vi "Calibration.vi"(8 "Error in":errorcluster) -> (0 "Error out":errorcluster)   [LabVIEW 2022 SP3, in "Bontech Calibration.lvlib" / "Bontech Calibration.lvclass"]
uses:
  Bontech Calibration.lvclass
  TypeDef/Calibration VI States.ctl
  Bontech Calibration.lvclass/Bontech Calibration.ctl
  <vilib>/vision/Image Controls.llb/IMAQ Image.ctl
  BonTechDetector/Controls/Acquisition Modes.ctl
  BonTechDetector/Controls/Acquisition Commands.ctl
  BonTechDetector/BonTechDetector.lvlib
panel:
  in  "Calibrate":bool
  in  "Get Bright Image":bool
  in  "Get Dark Image":bool
  out "Status":string
  out "Progress":u16(slide) scale=0.0..100.0
  # "Aayvu Calibration Tool"
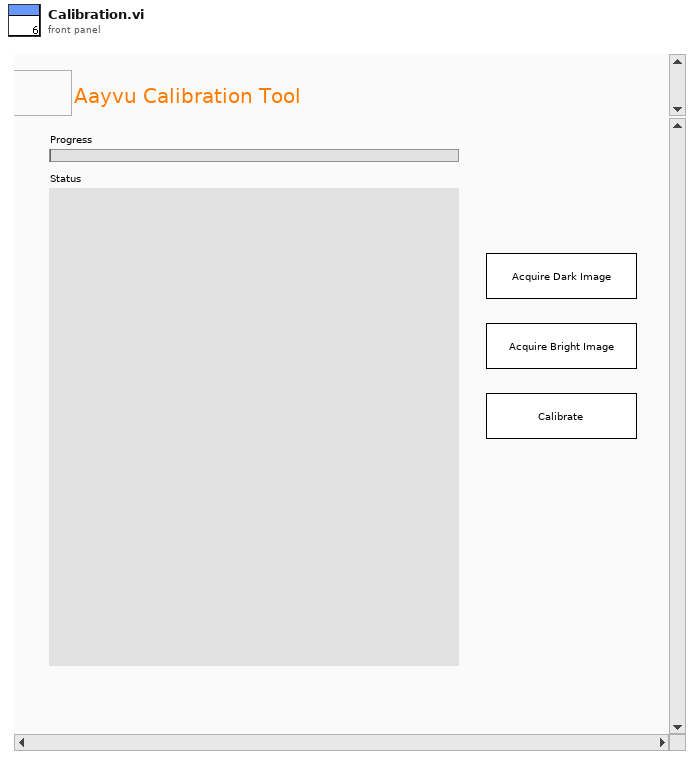
[diagram p1: front panel]
types:
  T1 = typedef "IMAQ Image.ctl" = refnum<image>
  T2 = cluster{"Status":string, "nWidth":u32, "nHeight":u32, "Save Path":string, "nSensorIP":string, "nHostIP":string, "live image":T1, "acq image":T1, "lpszSerialNum":string, "Progress":u8, "Iteration":i32, "refImg":u16[], "pImg":u16[], "Cal Dir":string, "avgBuff":dbl[], "pDarkImg":u16[], "pBrightImg":u16[]}
  T3 = cluster{"UI Ref":cluster{"Progress Ref":refnum<vi>, "Status Ref":refnum<vi>}, "Sensor Data":cluster{"nHostIP":string, "nSensorIP":string, "lpszSerialNum":string, "Cal Dir":string, "refImg":u16[], "pImg":u16[], "nHeight":u32, "nWidth":u32, "pBrightImg":u16[], "pDarkImg":u16[], "avgBuff":dbl[], "Iteration":i32, "Progress":u8, "acq image":T1, "live image":T1, "Save Path":string, "Status":string}}
  T4 = cluster{"Command":string, "Img Save Path":path, "pImg":u16[], "Iteration":i32, "Status":string}
  T5 = typedef "Calibration VI States.ctl" = enum16{"Poll", "Init", "Start Acquisition", "Acquire Dark Image", "Acquire Bright Image", "Calibrate", "Stop Acquisition", "Save Image", "Error", "Exit"}
  T6 = cluster{"nHostIP":string, "nSensorIP":string, "lpszSerialNum":string, "Cal Dir":string, "refImg":u16[], "pImg":u16[], "nHeight":u32, "nWidth":u32, "pBrightImg":u16[], "pDarkImg":u16[], "avgBuff":dbl[], "Iteration":i32, "Progress":u8, "acq image":T1, "live image":T1, "Save Path":string, "Status":string}
  T7 = typedef "BonTechDetector.lvlib/Acquisition Modes.ctl" = enum32{"IMAGECAP_TRIGGER_MODE", "IMAGECAP_AED_MODE", "IMAGECAP_SOFTTRIGGER_MODE", "IMAGECAP_AVG_COUNT_MODE", "IMAGECAP_AVG_AED_MODE", "IMAGECAP_CONTINUOUS_MODE", "IMAGECAP_VIEWER_MODE", "IMAGECAP_CONTINUOUS_BINNING_MODE"}
  T8 = typedef "Image Type" = u32
  T9 = typedef "BonTechDetector.lvlib/Acquisition Commands.ctl" = u32
  T10 = enum16{"big-endian, network order", "native, host order", "little-endian"}
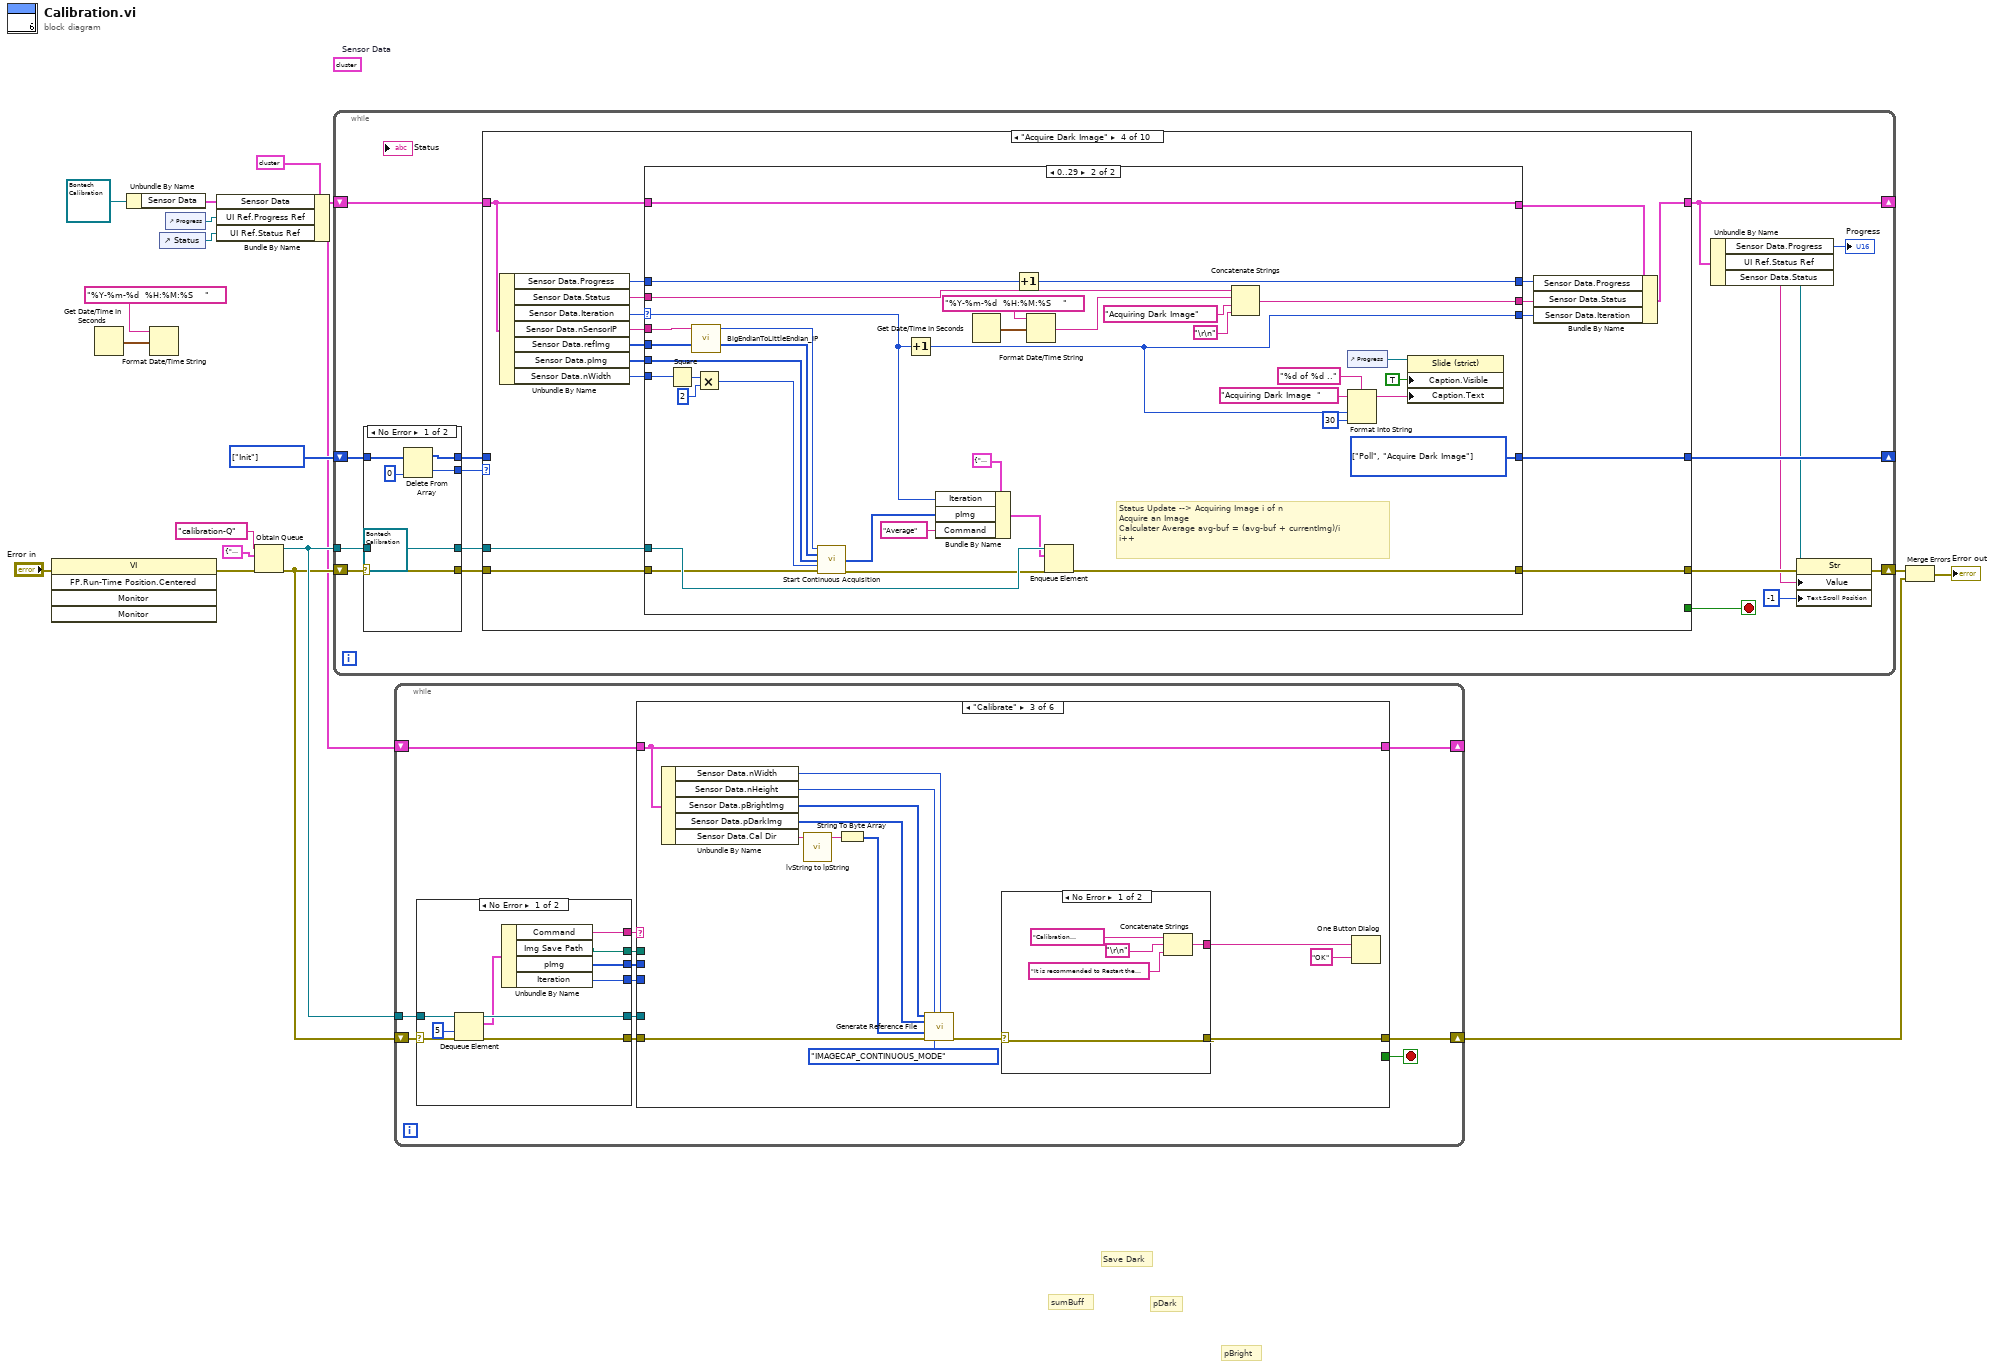
[diagram p0: block diagram]
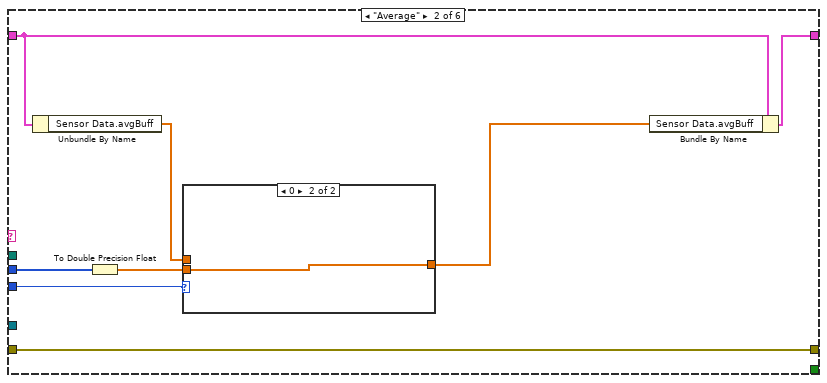
[diagram p3: hidden frame]
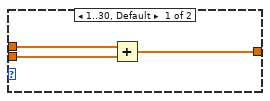
[diagram p4: hidden frame]
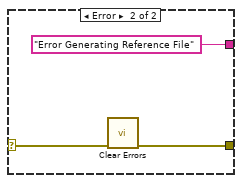
[diagram p5: hidden frame]
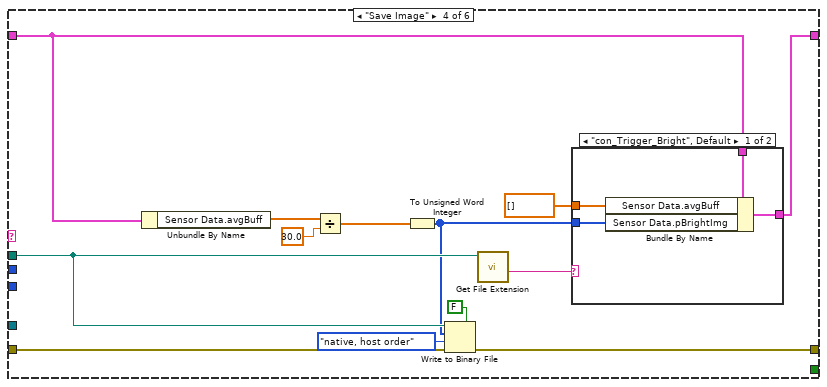
[diagram p6: hidden frame]
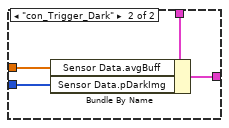
[diagram p7: hidden frame]
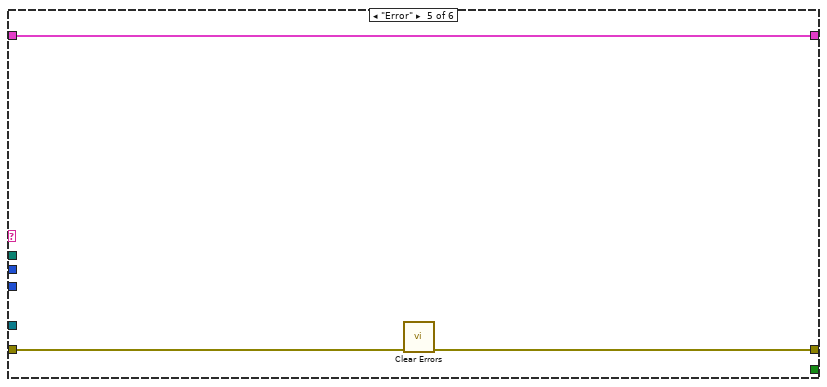
[diagram p8: hidden frame]
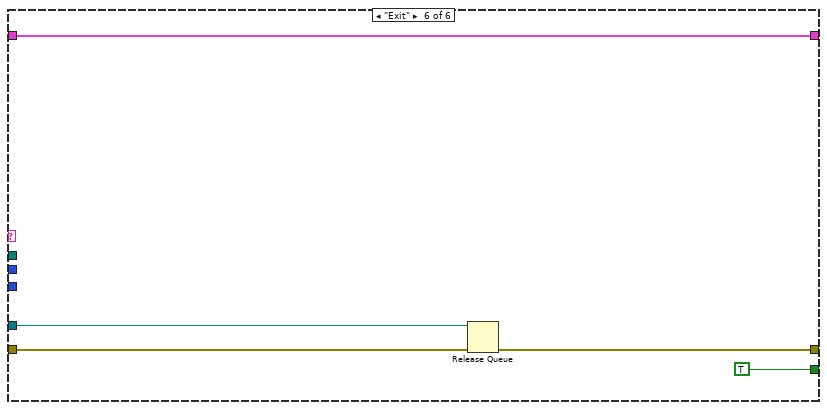
[diagram p9: hidden frame]
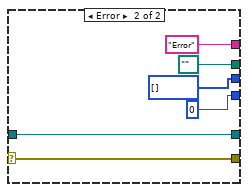
[diagram p10: hidden frame]
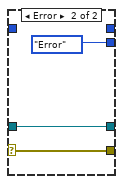
[diagram p11: hidden frame]
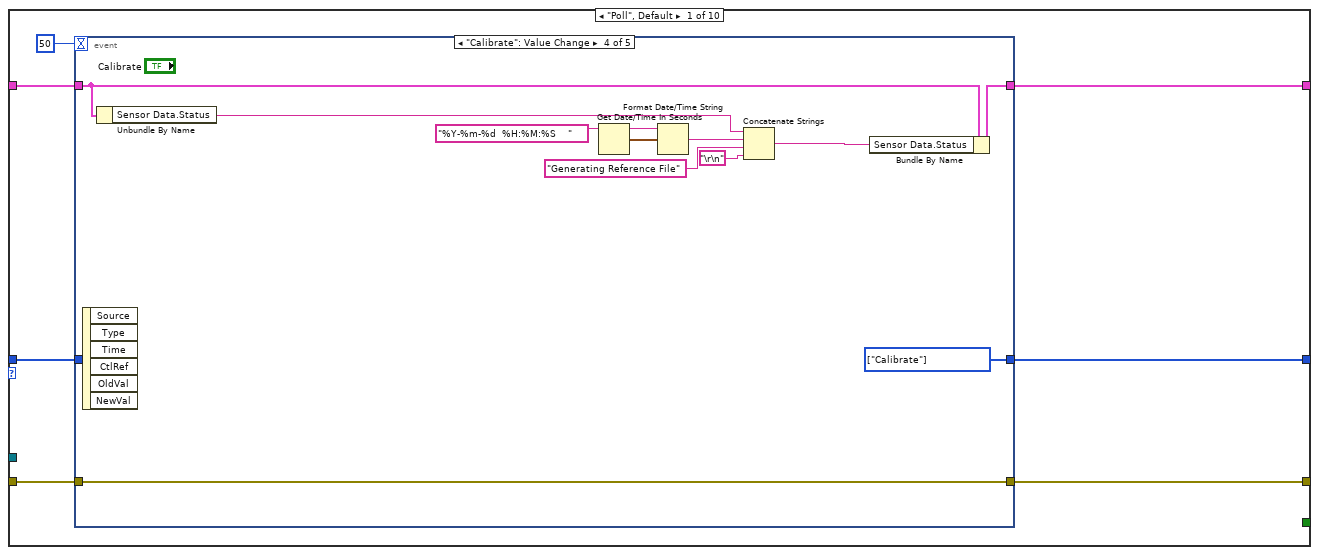
[diagram p12: hidden frame]
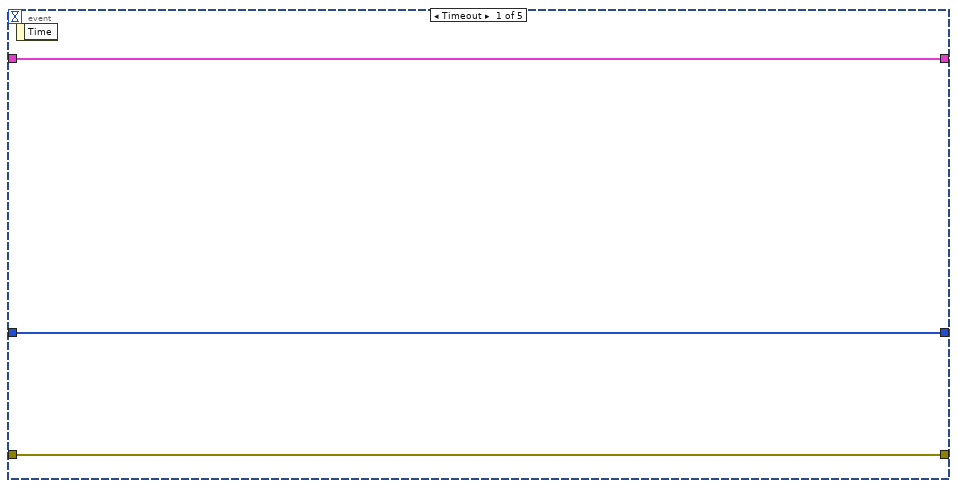
[diagram p13: hidden frame]
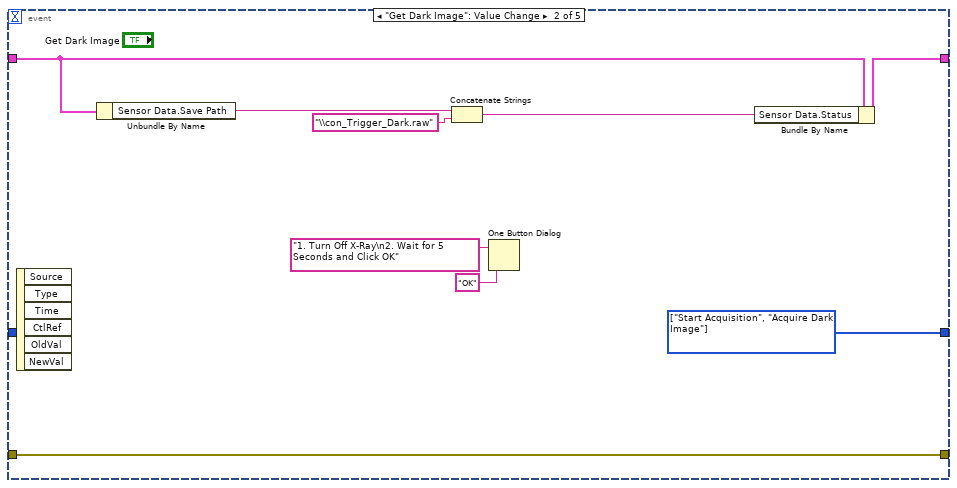
[diagram p14: hidden frame]
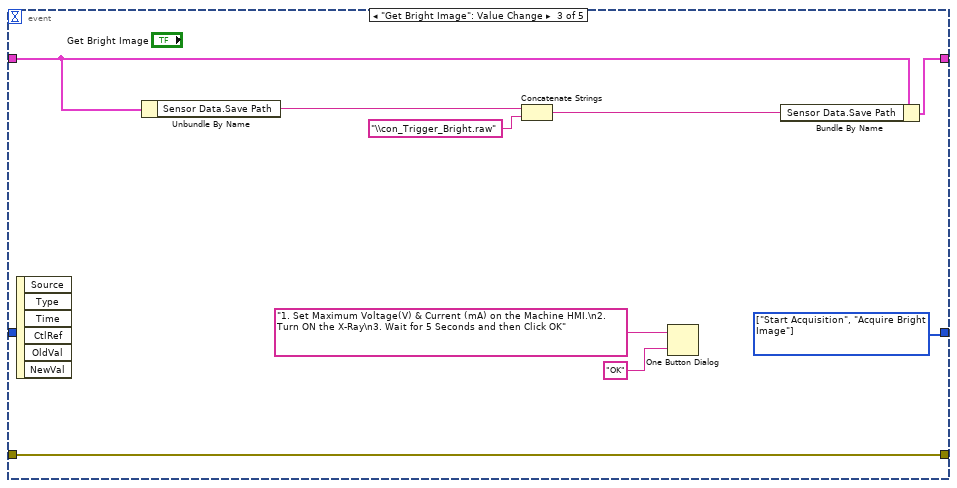
[diagram p15: hidden frame]
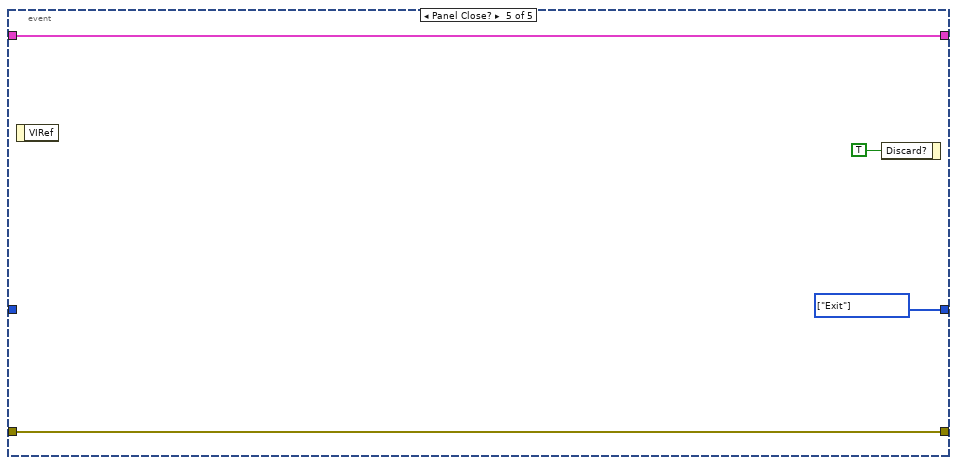
[diagram p16: hidden frame]
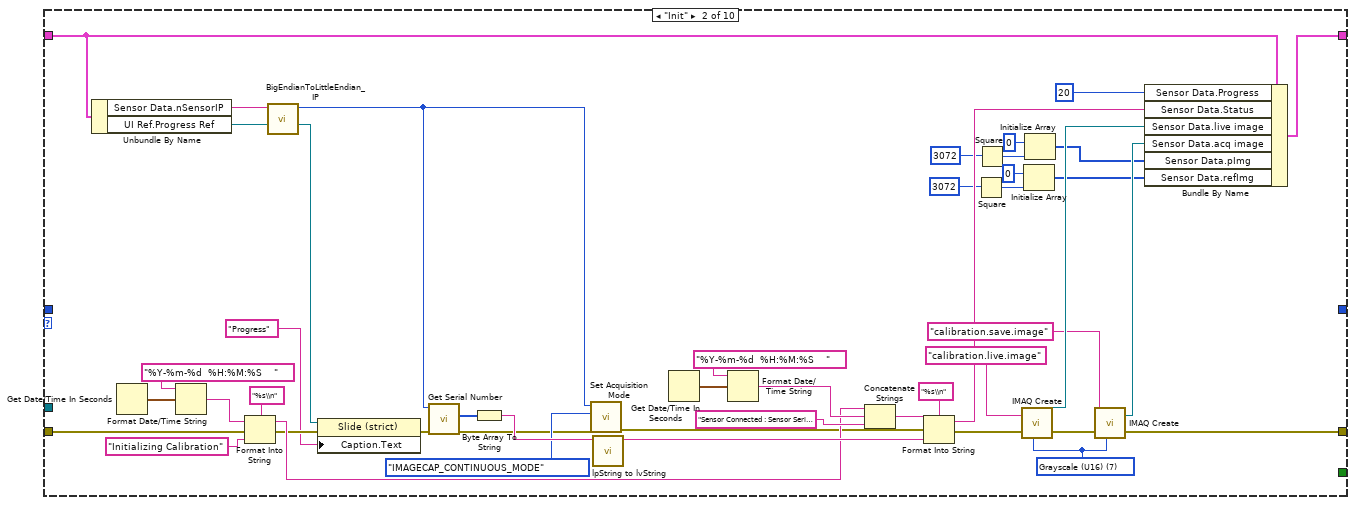
[diagram p17: hidden frame]
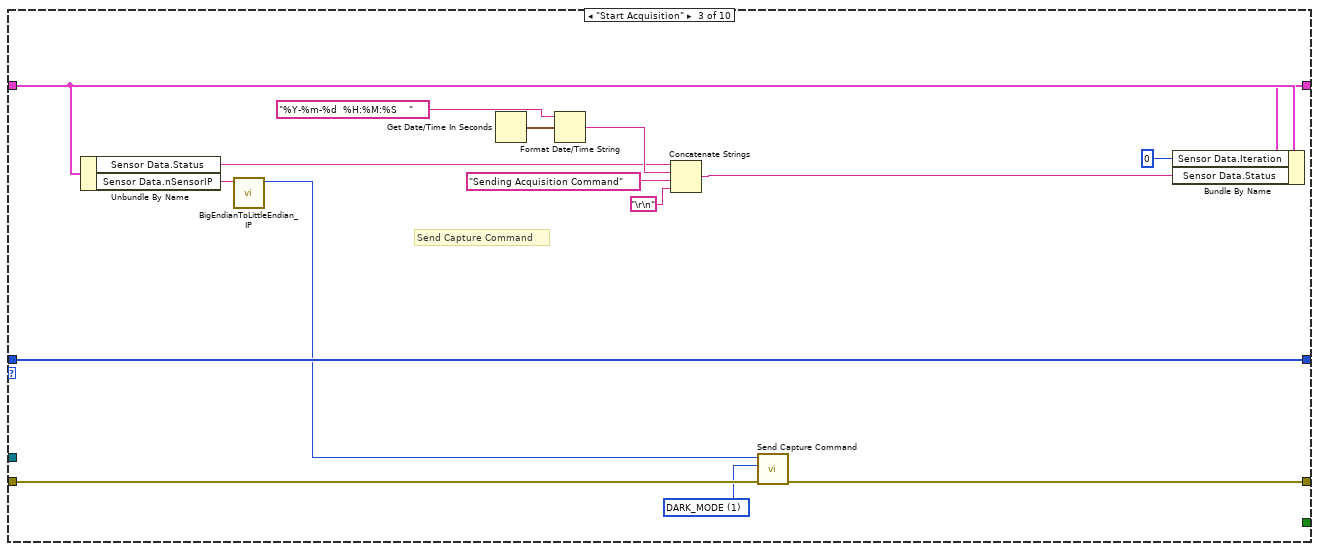
[diagram p18: hidden frame]
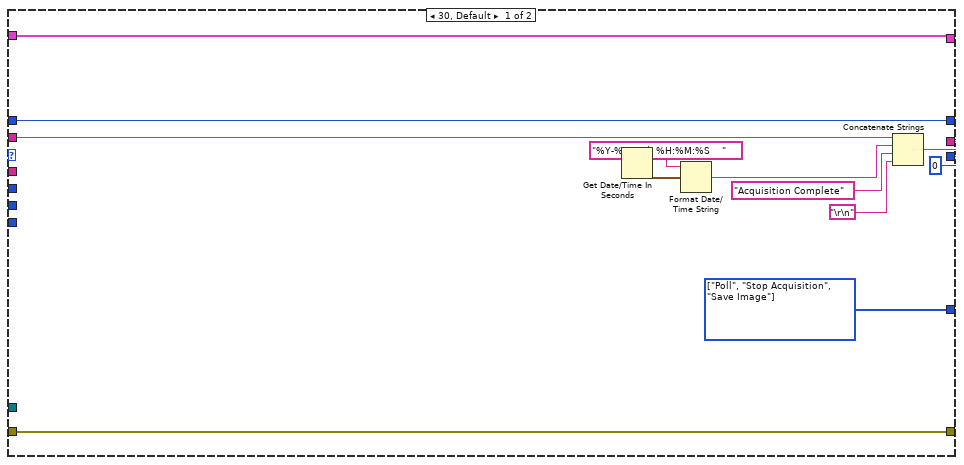
[diagram p19: hidden frame]
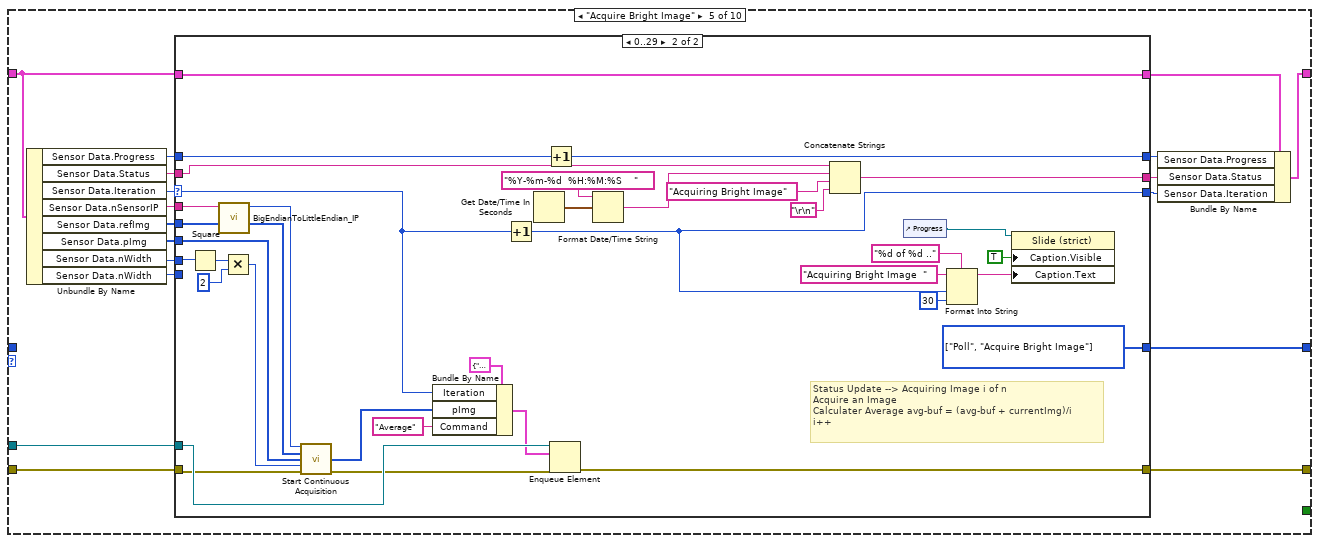
[diagram p20: hidden frame]
diagram:
  (unwired) T2 {"Status"="", "nWidth"=3072, "nHeight"=3072, "Save Path"="C:\\BSD\\192.168.3.240\\Reference", "nSensorIP"="192.168.3.240", "nHostIP"="192.168.3.5", "live image"=refnum, "acq image"=refnum, "lpszSerialNum"="", "Progress"=0, "Iteration"=0, "refImg"=[], "pImg"=[], "Cal Dir"="C:\\\\BSD\\\\192.168.3.240\\\\Reference", "avgBuff"=[], "pDarkImg"=[], "pBrightImg"=[]}  # Sensor Data
  w17 = T5[] [enum."Init"] items=["Poll", "Init", "Start Acquisition", "Acquire Dark Image", "Acquire Bright Image", "Calibrate", "Stop Acquisition", "Save Image", "Error", "Exit"]
  (unwired) refnum<class "Bontech Calibration.lvclass"> refnum ("Bontech Calibration.lvlib:Bontech Calibration.lvclass")
  # "Save Dark"
  # "pBright"
  # "pDark"
  # "sumBuff"
  n1 = invoke class="VI" method="FP.Run-Time Position.Centered"(error in="Error in") -> (error out=w10:errorcluster)  [unwired: 4 in, 4 out]
  n2 = Get Date/Time In Seconds() -> (seconds since 1Jan1904=w1:timestamp)
  n3 = Unbundle By Name(refnum<class "Bontech Calibration.lvclass"> refnum ("Bontech Calibration.lvlib:Bontech Calibration.lvclass")) -> ("Sensor Data"=w5:T6)
  n4 = Format Date/Time String(time format string (%c)="%Y-%m-%d  %H:%M:%S    ", seconds (now)=w1) -> ()  [unwired: 1 in, 1 out]
  n5 = control-ref of="Status"() -> (w3:refnum<vi>)
  n6 = control-ref of="Progress"() -> (w4:refnum<vi>)
  n7 = Bundle By Name(cluster=T3 {"UI Ref"={"Progress Ref"=refnum, "Status Ref"=refnum}, "Sensor Data"={"nHostIP"="", "nSensorIP"="", "lpszSerialNum"="", "Cal Dir"="", "refImg"=[], "pImg"=[], "nHeight"=0, "nWidth"=0, "pBrightImg"=[], "pDarkImg"=[], "avgBuff"=[], "Iteration"=0, "Progress"=0, "acq image"=refnum, "live image"=refnum, "Save Path"="", "Status"=""}}, "Sensor Data"=w5, "UI Ref.Progress Ref"=w4, "UI Ref.Status Ref"=w3) -> (w7:T3)
  n8 = Obtain Queue(name (unnamed)="calibration-Q", element data type=T4 {"Command"="", "Img Save Path"=path "", "pImg"=[], "Iteration"=0, "Status"=""}, error in (no error)=w10) -> (queue out=w13:refnum<queue>, error out=w9:errorcluster)  [unwired: 2 in, 1 out]
  n9 = while {
    shift-right: [w22] -> w18
    shift-left: w9 -> [w35]
    shift-right: [w28] -> _
    shift-left: w17 -> [w32]
    shift-right: [w26] -> _
    shift-left: w7 -> [w27]
    tunnel: w13 -> [w25]
    stop <- w29 stop-if-true
    n10 = case shown="No Error" w35 {
      selector: w35 -> [w41 w44]
      tunnel: [w41 w44] -> w34
      tunnel: w32 -> [w40 _]
      tunnel: [w38 _] -> w31
      tunnel: [w37 Calibration_VI_States."Error" ("Enum")] -> w30
      tunnel: w25 -> [w36 w42]
      tunnel: [w36 w42] -> w24
      frame No Error {
        n11 = Delete From Array(array=w40, index=0) -> (deleted portion=w37:T5, array with subset deleted=w38:T5[])  [unwired: 1 in]
      }
      frame Error {
      }
    }
    n12 = case shown="\"Acquire Dark Image\"" w30 {
      tunnel: w34 -> [w51 w110 w135 w164 w229 w279 w296 w306 w310 w325]
      tunnel: [w50 w88 w134 w163 w228 w281 w295 w305 w311 w313] -> w33
      tunnel: w31 -> [w47 _ w137 _ _ _ w299 _ _ _]
      tunnel: [_ _ _ _ _ _ _ _ _ TRUE] -> w29
      tunnel: [w48 _ w137 w165 w230 _ w299 _ _ _] -> w28
      tunnel: w27 -> [w46 w117 w148 w150 w213 w284 w298 w300 w312 w323]
      tunnel: [w45 w130 w146 w157 w221 w288 w298 w308 w312 w322] -> w26
      tunnel: w24 -> [_ _ _ w154 w218 w286 _ w304 _ w317]
      frame "Poll", Default {
        n13 = event shown="[3] \"Calibrate\": Value Change" {
          selector: _ -> [_ _ _ _ _]
          dyn-events: _ -> [_ _ _ _ _]
          timeout: 50 -> [_ _ _ _ _]
          tunnel: w51 -> [w54 w63 w72 w82 w84]
          tunnel: [w54 w63 w72 w82 w84] -> w50
          tunnel: [w53 w62 w71 w83 w86] -> w48
          tunnel: w47 -> [w53 _ _ _ _]
          tunnel: w46 -> [w52 w59 w65 w75 w85]
          tunnel: [w52 w56 w64 w74 w85] -> w45
          event Timeout {
            n14 = event-data() -> ()  [unwired: 1 in, 1 out]
          }
          event "Get Dark Image": Value Change {
            w62 = T5[] [enum."Start Acquisition", enum."Acquire Dark Image"] items=["Poll", "Init", "Start Acquisition", "Acquire Dark Image", "Acquire Bright Image", "Calibrate", "Stop Acquisition", "Save Image", "Error", "Exit"]
            n15 = event-data() -> ()  [unwired: 1 in, 6 out]
            n16 = Unbundle By Name(w59) -> ("Sensor Data.Save Path"=w58:string)
            n17 = Concatenate Strings(w58, "\\con_Trigger_Dark.raw" ("string")) -> (w55:string)
            n18 = One Button Dialog(message="1. Turn Off X-Ray\n2. Wait for 5 Seconds and Click OK", button name ("OK")="OK") -> ()  [unwired: 1 out]
            n19 = Bundle By Name(cluster=w59, "Sensor Data.Status"=w55) -> (w56:T3)
          }
          event "Get Bright Image": Value Change {
            w71 = T5[] [enum."Start Acquisition", enum."Acquire Bright Image"] items=["Poll", "Init", "Start Acquisition", "Acquire Dark Image", "Acquire Bright Image", "Calibrate", "Stop Acquisition", "Save Image", "Error", "Exit"]
            n20 = event-data() -> ()  [unwired: 1 in, 6 out]
            n21 = Unbundle By Name(w65) -> ("Sensor Data.Save Path"=w68:string)
            n22 = Concatenate Strings(w68, "\\con_Trigger_Bright.raw" ("string")) -> (w66:string)
            n23 = One Button Dialog(message="1. Set Maximum Voltage(V) & Current (mA) on the Machine HMI.\n2. Turn ON the X-Ray\n3. Wait for 5 Seconds and then Click OK", button name ("OK")="OK") -> ()  [unwired: 1 out]
            n24 = Bundle By Name(cluster=w65, "Sensor Data.Save Path"=w66) -> (w64:T3)
          }
          event "Calibrate": Value Change {
            w83 = T5[] [enum."Calibrate"] items=["Poll", "Init", "Start Acquisition", "Acquire Dark Image", "Acquire Bright Image", "Calibrate", "Stop Acquisition", "Save Image", "Error", "Exit"]
            n25 = event-data() -> ()  [unwired: 1 in, 6 out]
            n26 = Unbundle By Name(w75) -> ("Sensor Data.Status"=w76:string)
            n27 = Get Date/Time In Seconds() -> (seconds since 1Jan1904=w81:timestamp)
            n28 = Format Date/Time String(time format string (%c)="%Y-%m-%d  %H:%M:%S    ", seconds (now)=w81) -> (date/time string=w79:string)  [unwired: 1 in]
            n29 = Concatenate Strings(w76, w79, "Generating Reference File" ("string"), "\r\n") -> (w73:string)
            n30 = Bundle By Name(cluster=w75, "Sensor Data.Status"=w73) -> (w74:T3)
          }
          event Panel Close? {
            w86 = T5[] [enum."Exit"] items=["Poll", "Init", "Start Acquisition", "Acquire Dark Image", "Acquire Bright Image", "Calibrate", "Stop Acquisition", "Save Image", "Error", "Exit"]
            n31 = event-data() -> ()  [unwired: 1 in, 1 out]
            n32 = event-data("Discard?"=TRUE) -> ()  [unwired: 1 in, 1 out]
          }
        }
      }
      frame "Init" {
        w127 = T8 7 items=["Grayscale (U8)", "Grayscale (I16)", "Grayscale (SGL)", "Complex (CSG)", "RGB (U32)", "HSL (U32)", "RGB (U64)", "Grayscale (U16)"] ("Image Type")
        n33 = Unbundle By Name(w117) -> ("Sensor Data.nSensorIP"=w116:string, "UI Ref.Progress Ref"=w90:refnum<vi>)
        n34 = Get Date/Time In Seconds() -> (seconds since 1Jan1904=w114:timestamp)
        n35 = Format Date/Time String(time format string (%c)="%Y-%m-%d  %H:%M:%S    ", seconds (now)=w114) -> (date/time string=w112:string)  [unwired: 1 in]
        n36 = Format Into String(format string="%s\\n", initial string=w112, error in=w110, "Initializing Calibration" ("input 1")) -> (resulting string=w109:string, error out=w96:errorcluster)
        n37 = call "BigEndianToLittleEndian_IP.vi"("IP String"=w116) -> ("IP Network Order"=w92:u32)  [unwired: 10 in]
        n38 = property class="Slide (strict)"(reference=w90, error in=w96, "Caption.Text"="Progress") -> (error out=w91:errorcluster)  [unwired: 1 out]
        n39 = call "Get Serial Number.vi"("error in (no error)"=w91, "nSensorIP"=w92) -> ("error out"=w94:errorcluster, "lpszSerialNum out"=w97:u8[])  [unwired: 7 in, 1 out]
        n40 = Byte Array To String(unsigned byte array=w97) -> (string=w106:string)
        n41 = call "Set Acquisition Mode.vi"("error in (no error)"=w94, "nMode"=Acquisition_Modes."IMAGECAP_CONTINUOUS_MODE", "nSensorIP"=w92) -> ("error out"=w93:errorcluster)  [unwired: 7 in, 1 out]
        n42 = call "lpString to lvString.vi"("LPTSTR String"=w106) -> ("LVString"=w119:string)  [unwired: 10 in]
        n43 = Get Date/Time In Seconds() -> (seconds since 1Jan1904=w121:timestamp)
        n44 = Format Date/Time String(time format string (%c)="%Y-%m-%d  %H:%M:%S    ", seconds (now)=w121) -> (date/time string=w120:string)  [unwired: 1 in]
        n45 = Concatenate Strings(w109, w120, "Sensor Connected : Sensor Serial Number - " ("initial string")) -> (w123:string)
        n46 = Format Into String(format string="%s\\n", initial string=w123, error in=w93, w119) -> (resulting string=w115:string, error out=w118:errorcluster)
        n47 = Square(x=3072) -> (x^2=w100:i32)
        n48 = Square(x=3072) -> (x^2=w104:i32)
        n49 = call "IMAQ Create"("Image Name"="calibration.live.image", "Image Type"=w127, "error in (no error)"=w118) -> ("New Image"=w128:T1, "error out"=w132:errorcluster)  [unwired: 2 in]
        n50 = Initialize Array(u16 0 ("element"), w100) -> (w98:u16[])
        n51 = Initialize Array(u16 0 ("element"), w104) -> (w102:u16[])
        n52 = call "IMAQ Create"("Image Name"="calibration.save.image", "Image Type"=w127, "error in (no error)"=w132) -> ("New Image"=w129:T1, "error out"=w88:errorcluster)  [unwired: 2 in]
        n53 = Bundle By Name(cluster=w117, "Sensor Data.Progress"=u8 20 ("Progress"), "Sensor Data.Status"=w115, "Sensor Data.live image"=w128, "Sensor Data.acq image"=w129, "Sensor Data.pImg"=w102, "Sensor Data.refImg"=w98) -> (w130:T3)
      }
      frame "Start Acquisition" {
        w133 = T9 1 items=["ACQ_INIT"=0, "DARK_MODE"=1, "BRIGHT_MODE"=2, "SOFTTRIGGER_MODE"=258, "SOFTTRIGGER_INSTANT_MODE"=259] ("nCmd")
        # "Send Capture Command"
        n54 = Unbundle By Name(w148) -> ("Sensor Data.Status"=w139:string, "Sensor Data.nSensorIP"=w147:string)
        n55 = call "BigEndianToLittleEndian_IP.vi"("IP String"=w147) -> ("IP Network Order"=w136:u32)  [unwired: 10 in]
        n56 = Get Date/Time In Seconds() -> (seconds since 1Jan1904=w144:timestamp)
        n57 = Format Date/Time String(time format string (%c)="%Y-%m-%d  %H:%M:%S    ", seconds (now)=w144) -> (date/time string=w142:string)  [unwired: 1 in]
        n58 = Concatenate Strings(w139, w142, "Sending Acquisition Command" ("string"), "\r\n") -> (w140:string)
        n59 = call "Send Capture Command.vi"("error in (no error)"=w135, "nCmd"=w133, "nSensorIP"=w136) -> ("error out"=w134:errorcluster)  [unwired: 7 in, 1 out]
        n60 = Bundle By Name(cluster=w148, "Sensor Data.Iteration"=0 ("Iteration"), "Sensor Data.Status"=w140) -> (w146:T3)
      }
      frame "Acquire Dark Image" {
        n61 = Unbundle By Name(w150) -> ("Sensor Data.Progress"=w152:u8, "Sensor Data.Status"=w156:string, "Sensor Data.Iteration"=w162:i32, "Sensor Data.nSensorIP"=w161:string, "Sensor Data.refImg"=w160:u16[], "Sensor Data.pImg"=w159:u16[], "Sensor Data.nWidth"=w158:u32)
        n62 = case shown="0..29" w162 {
          selector: w162 -> [_ w201]
          tunnel: [w177 w212] -> w165
          tunnel: w164 -> [w176 w185]
          tunnel: [w176 w192] -> w163
          tunnel: w161 -> [_ w211]
          tunnel: w160 -> [_ w182]
          tunnel: w159 -> [_ w181]
          tunnel: w158 -> [_ w210]
          tunnel: [0 w191] -> w153
          tunnel: w156 -> [w169 w205]
          tunnel: [w171 w204] -> w155
          tunnel: w154 -> [_ w202]
          tunnel: w152 -> [w167 w199]
          tunnel: [w167 w195] -> w151
          tunnel: w150 -> [w166 w198]
          tunnel: [w166 w198] -> w149
          frame 30, Default {
            w177 = T5[] [enum."Poll", enum."Stop Acquisition", enum."Save Image"] items=["Poll", "Init", "Start Acquisition", "Acquire Dark Image", "Acquire Bright Image", "Calibrate", "Stop Acquisition", "Save Image", "Error", "Exit"]
            n63 = Get Date/Time In Seconds() -> (seconds since 1Jan1904=w173:timestamp)
            n64 = Format Date/Time String(time format string (%c)="%Y-%m-%d  %H:%M:%S    ", seconds (now)=w173) -> (date/time string=w170:string)  [unwired: 1 in]
            n65 = Concatenate Strings(w169, w170, "Acquisition Complete", "\r\n") -> (w171:string)
          }
          frame 0..29 {
            w212 = T5[] [enum."Poll", enum."Acquire Dark Image"] items=["Poll", "Init", "Start Acquisition", "Acquire Dark Image", "Acquire Bright Image", "Calibrate", "Stop Acquisition", "Save Image", "Error", "Exit"]
            # "Status Update --> Acquiring Image i of n\nAcquire an Image\nCalculater Average avg-buf = (avg-buf + currentImg)/i\ni++"
            n66 = Square(x=w210) -> (x^2=w187:u32)
            n67 = call "BigEndianToLittleEndian_IP.vi"("IP String"=w211) -> ("IP Network Order"=w183:u32)  [unwired: 10 in]
            n68 = Multiply(x=w187, y=2 ("value")) -> (x*y=w180:u32)
            n69 = call "Start Continuous Acquisition.vi"("nSensorIP"=w183, "refImg"=w182, "pImg"=w181, "nBuffLength"=w180, "error in (no error)"=w185) -> ("pImg out"=w179:u16[], "error out"=w184:errorcluster)  [unwired: 7 in, 2 out]
            n70 = Increment(x=w201) -> (x+1=w191:i32)
            n71 = Bundle By Name(cluster=T4 {"Command"="", "Img Save Path"=path "", "pImg"=[], "Iteration"=0, "Status"=""}, "Iteration"=w201, "pImg"=w179, "Command"="Average") -> (w196:T4)
            n72 = Get Date/Time In Seconds() -> (seconds since 1Jan1904=w209:timestamp)
            n73 = Increment(x=w199) -> (x+1=w195:u8)
            n74 = Format Date/Time String(time format string (%c)="%Y-%m-%d  %H:%M:%S    ", seconds (now)=w209) -> (date/time string=w207:string)  [unwired: 1 in]
            n75 = Enqueue Element(queue=w202, element=w196, error in (no error)=w184) -> (error out=w192:errorcluster)  [unwired: 1 in, 2 out]
            n76 = Concatenate Strings(w205, w207, "Acquiring Dark Image" ("string"), "\r\n") -> (w204:string)
            n77 = control-ref of="Progress"() -> (w178:refnum<vi>)
            n78 = Format Into String(format string="%d of %d ..", initial string="Acquiring Dark Image  ", w191, u8 30 ("input 2")) -> (resulting string=w189:string)  [unwired: 1 in, 1 out]
            n79 = property class="Slide (strict)"(reference=w178, "Caption.Visible"=TRUE, "Caption.Text"=w189) -> ()  [unwired: 1 in, 2 out]
          }
        }
        n80 = Bundle By Name(cluster=w149, "Sensor Data.Progress"=w151, "Sensor Data.Status"=w155, "Sensor Data.Iteration"=w153) -> (w157:T3)
      }
      frame "Acquire Bright Image" {
        n81 = Unbundle By Name(w213) -> ("Sensor Data.Progress"=w215:u8, "Sensor Data.Status"=w220:string, "Sensor Data.Iteration"=w227:i32, "Sensor Data.nSensorIP"=w226:string, "Sensor Data.refImg"=w225:u16[], "Sensor Data.pImg"=w224:u16[], "Sensor Data.nWidth"=w223:u32, "Sensor Data.nWidth"=w222:u32)
        n82 = case shown="0..29" w227 {
          selector: w227 -> [_ w265]
          tunnel: [w242 w277] -> w230
          tunnel: w229 -> [w241 w250]
          tunnel: [w241 w268] -> w228
          tunnel: w226 -> [_ w276]
          tunnel: w225 -> [_ w248]
          tunnel: w224 -> [_ w247]
          tunnel: w223 -> [_ w252]
          tunnel: w222 -> [_ _]
          tunnel: [0 w254] -> w217
          tunnel: w220 -> [w234 w271]
          tunnel: [w236 w270] -> w219
          tunnel: w218 -> [_ w267]
          tunnel: [w232 w262] -> w216
          tunnel: w215 -> [w232 w263]
          tunnel: w213 -> [w231 w261]
          tunnel: [w231 w261] -> w214
          frame 30, Default {
            w242 = T5[] [enum."Poll", enum."Stop Acquisition", enum."Save Image"] items=["Poll", "Init", "Start Acquisition", "Acquire Dark Image", "Acquire Bright Image", "Calibrate", "Stop Acquisition", "Save Image", "Error", "Exit"]
            n83 = Get Date/Time In Seconds() -> (seconds since 1Jan1904=w238:timestamp)
            n84 = Format Date/Time String(time format string (%c)="%Y-%m-%d  %H:%M:%S    ", seconds (now)=w238) -> (date/time string=w235:string)  [unwired: 1 in]
            n85 = Concatenate Strings(w234, w235, "Acquisition Complete", "\r\n") -> (w236:string)
          }
          frame 0..29 {
            w277 = T5[] [enum."Poll", enum."Acquire Bright Image"] items=["Poll", "Init", "Start Acquisition", "Acquire Dark Image", "Acquire Bright Image", "Calibrate", "Stop Acquisition", "Save Image", "Error", "Exit"]
            # "Status Update --> Acquiring Image i of n\nAcquire an Image\nCalculater Average avg-buf = (avg-buf + currentImg)/i\ni++"
            n86 = Square(x=w252) -> (x^2=w251:u32)
            n87 = call "BigEndianToLittleEndian_IP.vi"("IP String"=w276) -> ("IP Network Order"=w249:u32)  [unwired: 10 in]
            n88 = Multiply(x=w251, y=2 ("value")) -> (x*y=w246:u32)
            n89 = call "Start Continuous Acquisition.vi"("nSensorIP"=w249, "refImg"=w248, "pImg"=w247, "nBuffLength"=w246, "error in (no error)"=w250) -> ("pImg out"=w244:u16[], "error out"=w245:errorcluster)  [unwired: 7 in, 2 out]
            n90 = Bundle By Name(cluster=T4 {"Command"="", "Img Save Path"=path "", "pImg"=[], "Iteration"=0, "Status"=""}, "Iteration"=w265, "pImg"=w244, "Command"="Average") -> (w266:T4)
            n91 = Increment(x=w265) -> (x+1=w254:i32)
            n92 = Get Date/Time In Seconds() -> (seconds since 1Jan1904=w275:timestamp)
            n93 = Increment(x=w263) -> (x+1=w262:u8)
            n94 = Enqueue Element(queue=w267, element=w266, error in (no error)=w245) -> (error out=w268:errorcluster)  [unwired: 1 in, 2 out]
            n95 = Format Date/Time String(time format string (%c)="%Y-%m-%d  %H:%M:%S    ", seconds (now)=w275) -> (date/time string=w273:string)  [unwired: 1 in]
            n96 = Concatenate Strings(w271, w273, "Acquiring Bright Image" ("string"), "\r\n") -> (w270:string)
            n97 = control-ref of="Progress"() -> (w243:refnum<vi>)
            n98 = Format Into String(format string="%d of %d ..", initial string="Acquiring Bright Image  ", w254, u8 30 ("input 2")) -> (resulting string=w256:string)  [unwired: 1 in, 1 out]
            n99 = property class="Slide (strict)"(reference=w243, "Caption.Visible"=TRUE, "Caption.Text"=w256) -> ()  [unwired: 1 in, 2 out]
          }
        }
        n100 = Bundle By Name(cluster=w214, "Sensor Data.Progress"=w216, "Sensor Data.Status"=w219, "Sensor Data.Iteration"=w217) -> (w221:T3)
      }
      frame "Calibrate" {
        n101 = property on="Progress" class="Slide (strict)"(error in=w279, "Caption.Text"="Generating Reference File") -> (error out=w278:errorcluster)  [unwired: 1 in, 1 out]
        n102 = Bundle By Name(cluster=T4 {"Command"="", "Img Save Path"=path "", "pImg"=[], "Iteration"=0, "Status"=""} ("element"), "Command"="Calibrate") -> (w283:T4)
        n103 = Enqueue Element(queue=w286, element=w283, error in (no error)=w278) -> (error out=w281:errorcluster)  [unwired: 1 in, 2 out]
        n104 = disable-structure shown="Disabled" {
          disable-tunnel: [w293 _] -> _
          frame Disabled {
            n105 = Get Date/Time In Seconds() -> (seconds since 1Jan1904=w292:timestamp)
            n106 = Format Date/Time String(time format string (%c)="%Y-%m-%d  %H:%M:%S    ", seconds (now)=w292) -> (date/time string=w290:string)  [unwired: 1 in]
            n107 = Concatenate Strings(w290, "\r\n") -> (w293:string)  [unwired: 2 in]
          }
          frame Enabled {
          }
        }
        n108 = Bundle By Name(cluster=w284, "Sensor Data.Progress"=u8 100 ("Progress")) -> (w288:T3)
      }
      frame "Stop Acquisition" {
        # "Send StopContinuousAcquisition"
        n109 = Unbundle By Name(w298) -> ("Sensor Data.nSensorIP"=w297:string)
        n110 = call "BigEndianToLittleEndian_IP.vi"("IP String"=w297) -> ("IP Network Order"=w294:u32)  [unwired: 10 in]
        n111 = call "Stop Continuous Acquisition.vi"("error in (no error)"=w296, "nSensorIP"=w294) -> ("error out"=w295:errorcluster)  [unwired: 8 in, 1 out]
      }
      frame "Save Image" {
        # "Save the array as binary file."
        n112 = Bundle By Name(cluster=T4 {"Command"="", "Img Save Path"=path "", "pImg"=[], "Iteration"=0, "Status"=""}, "Command"="Save Image") -> (w303:T4)
        n113 = Enqueue Element(queue=w304, element=w303, error in (no error)=w306) -> (error out=w305:errorcluster)  [unwired: 1 in, 2 out]
        n114 = Bundle By Name(cluster=w300, "Sensor Data.Iteration"=0 ("Iteration")) -> (w308:T3)
      }
      frame "Error" {
        n115 = call <vilib>:"Simple Error Handler.vi"("error in (no error)"=w310) -> ("error out"=w309:errorcluster)  [unwired: 4 in, 4 out]
        n116 = call <vilib>:"Clear Errors.vi"("error in (no error)"=w309) -> ("error out"=w311:errorcluster)  [unwired: 5 in, 1 out]
      }
      frame "Exit" {
        n117 = Flush Queue(queue=w317, error in (no error)=w325) -> (queue out=w318:refnum<queue>, error out=w319:errorcluster)  [unwired: 1 out]
        n118 = Bundle By Name(cluster=T4 {"Command"="", "Img Save Path"=path "", "pImg"=[], "Iteration"=0, "Status"=""}, "Command"="Exit") -> (w316:T4)
        n119 = Enqueue Element At Opposite End(queue=w318, element=w316, error in (no error)=w319) -> (error out=w313:errorcluster)  [unwired: 1 in, 2 out]
        n120 = Bundle By Name(cluster=w323, "Sensor Data.Status"="" ("Status"), "Sensor Data.Progress"=u8 0 ("Progress")) -> (w322:T3)
      }
    }
    n121 = Unbundle By Name(w26) -> ("Sensor Data.Progress"=→"Progress":u8, "UI Ref.Status Ref"=w21:refnum<vi>, "Sensor Data.Status"=w20:string)
    n122 = property class="Str"(reference=w21, error in=w33, "Value"=w20, "Text.Scroll Position"=-1 ("count (1)")) -> (error out=w22:errorcluster)  [unwired: 1 out]
  }
  n123 = while {
    shift-right: [w335] -> w11
    shift-left: w9 -> [w337]
    tunnel: w13 -> [w334]
    shift-right: [w326] -> _
    shift-left: w7 -> [w327]
    stop <- w333 stop-if-true
    n124 = case shown="No Error" w337 {
      selector: w337 -> [w412 w417]
      tunnel: [w411 w417] -> w336
      tunnel: w334 -> [w410 w418]
      tunnel: [w409 w418] -> w331
      tunnel: [w407 "Error" ("Command")] -> w332
      tunnel: [w406 0 ("Iteration")] -> w330
      tunnel: [w405 u16[] [] ("pImg")] -> w329
      tunnel: [w404 path "" ("Img Save Path")] -> w328
      frame No Error {
        n125 = Dequeue Element(queue=w410, timeout in ms (-1)=5, error in (no error)=w412) -> (queue out=w409:refnum<queue>, element=w408:T4, error out=w411:errorcluster)  [unwired: 1 out]
        n126 = Unbundle By Name(w408) -> ("Command"=w407:string, "Img Save Path"=w404:path, "pImg"=w405:u16[], "Iteration"=w406:i32)
      }
      frame Error {
      }
    }
    n127 = case shown="\"Calibrate\"" w332 {
      tunnel: [w339 w347 w361 w385 w395 w399] -> w335
      tunnel: w336 -> [w339 w347 w359 w386 w397 w400]
      tunnel: [_ _ _ _ _ TRUE] -> w333
      tunnel: w331 -> [_ _ _ _ _ w398]
      tunnel: w330 -> [_ w342 _ _ _ _]
      tunnel: w329 -> [_ w346 _ _ _ _]
      tunnel: w328 -> [_ _ _ w382 _ _]
      tunnel: w327 -> [w338 w345 w365 w380 w396 w401]
      tunnel: [w338 w343 w365 w379 w396 w401] -> w326
      frame "Poll", Default {
      }
      frame "Average" {
        n128 = Unbundle By Name(w345) -> ("Sensor Data.avgBuff"=w344:dbl[])
        n129 = To Double Precision Float(number=w346) -> (double precision float=w341:dbl[])
        n130 = case shown="0" w342 {
          tunnel: w341 -> [w350 w351]
          tunnel: [w348 w351] -> w340
          tunnel: w344 -> [w349 _]
          frame 1..30, Default {
            n131 = Add(x=w349, y=w350) -> (x+y=w348:dbl[])
          }
          frame 0 {
          }
        }
        n132 = Bundle By Name(cluster=w345, "Sensor Data.avgBuff"=w340) -> (w343:T3)
      }
      frame "Calibrate" {
        n133 = Unbundle By Name(w365) -> ("Sensor Data.nWidth"=w355:u32, "Sensor Data.nHeight"=w354:u32, "Sensor Data.pBrightImg"=w357:u16[], "Sensor Data.pDarkImg"=w356:u16[], "Sensor Data.Cal Dir"=w364:string)
        n134 = call "lvString to lpString.vi"("LVString"=w364) -> ("LPTSTR String"=w363:string)  [unwired: 10 in]
        n135 = String To Byte Array(string=w363) -> (unsigned byte array=w353:u8[])
        n136 = call "Generate Reference File.vi"("pBrightImage"=w357, "nWidth"=w354, "nHeight"=w355, "pDarkImage"=w356, "lpszSavePath"=w353, "error in"=w359, "Acquisition Mode"=Acquisition_Modes."IMAGECAP_CONTINUOUS_MODE") -> ("error out"=w358:errorcluster)  [unwired: 7 in, 1 out]
        n137 = case shown="No Error" w358 {
          selector: w358 -> [w368 w373]
          tunnel: [w368 w371] -> w361
          tunnel: [w370 "Error Generating Reference File" ("string")] -> w360
          frame No Error {
            n138 = Concatenate Strings("Calibration Complete.." ("string"), "\r\n", "It is recommended to Restart the application after the Calibration Process.." ("message")) -> (w370:string)
          }
          frame Error {
            n139 = call <vilib>:"Clear Errors.vi"("error in (no error)"=w373) -> ("error out"=w371:errorcluster)  [unwired: 5 in, 1 out]
          }
        }
        n140 = One Button Dialog(message=w360, button name ("OK")="OK") -> ()  [unwired: 1 out]
      }
      frame "Save Image" {
        n141 = Unbundle By Name(w380) -> ("Sensor Data.avgBuff"=w374:dbl[])
        n142 = Divide(x=w374, y=30.0) -> (x/y=w376:dbl[])
        n143 = To Unsigned Word Integer(number=w376) -> (unsigned 16bit integer=w377:u16[])
        n144 = Write to Binary File(file (use dialog)=w382, data=w377, error in=w386, 5:FALSE ("prepend array or string size? (T)"), 9:T10."native, host order" ("byte order (0:big-endian, network order)")) -> (error out=w385:errorcluster)  [unwired: 1 in, 2 out]
        n145 = call <vilib>:"Get File Extension.vi"("file"=w382) -> ("filename without extension"=w381:string)  [unwired: 6 in, 4 out]
        n146 = case shown="\"con_Trigger_Bright\", Default" w381 {
          tunnel: w380 -> [w389 w394]
          tunnel: [w390 w393] -> w379
          tunnel: dbl[] [] ("avgBuff") -> [w387 w392]
          tunnel: w377 -> [w388 w391]
          frame "con_Trigger_Bright", Default {
            n147 = Bundle By Name(cluster=w389, "Sensor Data.avgBuff"=w387, "Sensor Data.pBrightImg"=w388) -> (w390:T3)
          }
          frame "con_Trigger_Dark" {
            n148 = Bundle By Name(cluster=w394, "Sensor Data.avgBuff"=w392, "Sensor Data.pDarkImg"=w391) -> (w393:T3)
          }
        }
      }
      frame "Error" {
        n149 = call <vilib>:"Clear Errors.vi"("error in (no error)"=w397) -> ("error out"=w395:errorcluster)  [unwired: 5 in, 1 out]
      }
      frame "Exit" {
        n150 = Release Queue(queue=w398, error in (no error)=w400) -> (error out=w399:errorcluster)  [unwired: 1 in, 2 out]
      }
    }
  }
  n151 = Merge Errors(w18, w11) -> (→"Error out":errorcluster)
